vi "抽样与分割 - 副本.vi"(4 "stop (F)":bool caption="停止(F)", 8 "采样数":i32, 9 "采样率":i32[](array[numeric])=[32000, 32000, 32000, 32000, 32000, 32000, 80000, 80000], 10 "6133队列":refnum<queue>, 11 "数据队列":refnum<queue>) -> ()   [LabVIEW 2014]
panel:
  in  "发送次数":i32=1
  out "每通道发送的数据量":i32[](array[numeric])
  in  "读取次数":dbl=1.0
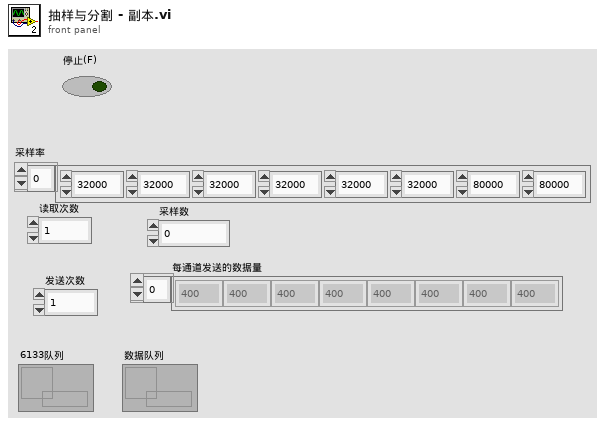
[diagram p1: front panel]
types:
  T1 = cluster{"设备名":string, "时间":timestamp, "数据":sgl[][]}
  T2 = cluster{"设备名":string, "时间":timestamp, "输出数组":dbl[][], "每通道发送的数据量":i32[], i32}
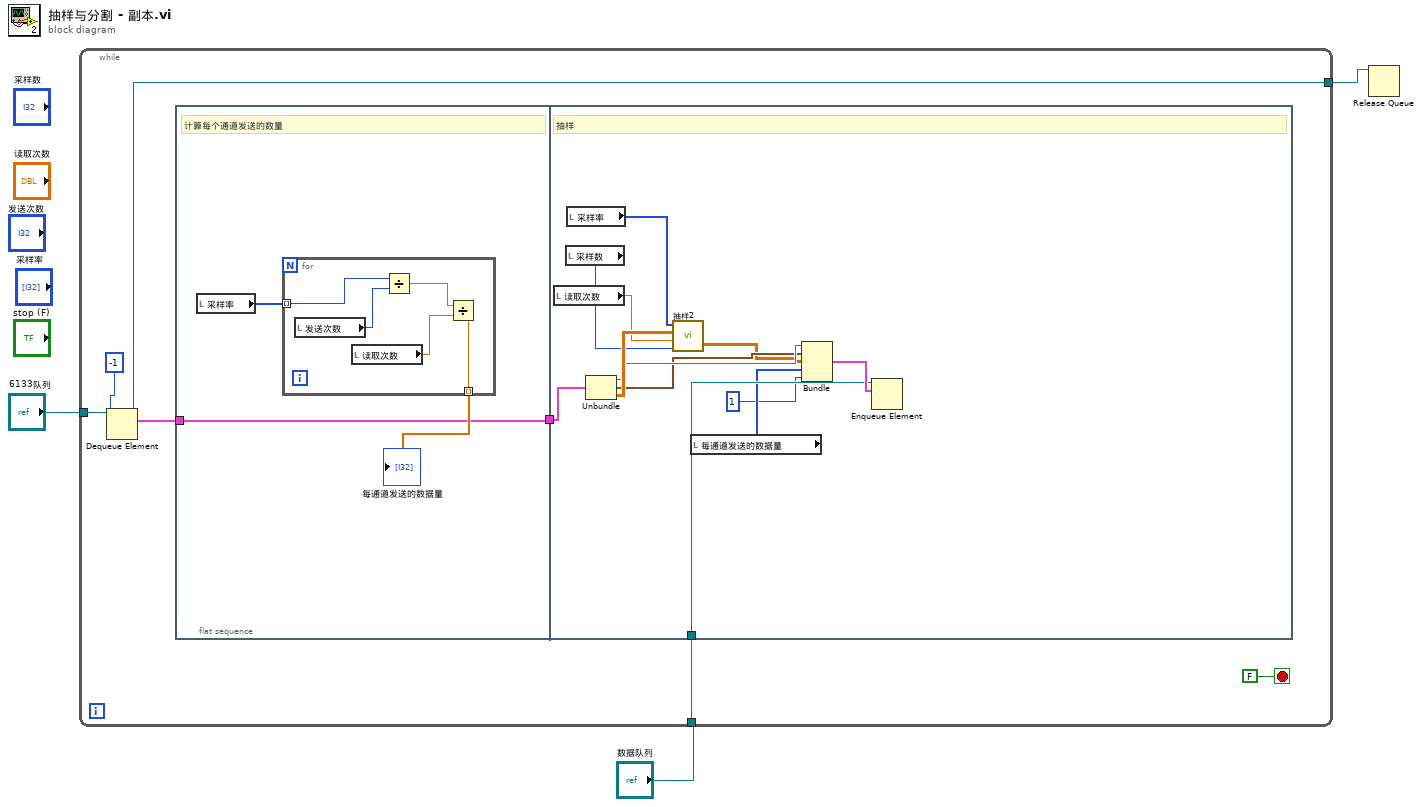
[diagram p0: block diagram]
diagram:
  n1 = while "While循环" {
    tunnel: "6133队列" -> [w10]
    tunnel: [w9] -> w2
    tunnel: "数据队列" -> [w4]
    stop <- FALSE stop-if-true
    n2 = Dequeue Element(queue=w10, timeout in ms (-1)=-1 ("超时毫秒(-1)")) -> (queue out=w9:refnum<queue>, element=w7:T1)  [unwired: 1 in, 2 out]
    n3 = flat-sequence "平铺式顺序结构" {
      tunnel: [w11] -> w6
      tunnel: w7 -> [w11]
      tunnel: w6 -> [w30]
      tunnel: w4 -> [w24]
      frame #0 {
        # "计算每个通道发送的数量"
        n4 = local read "采样率"() -> (w13:i32[])
        n5 = for "For循环" {
          tunnel: w13 -> [w15] mode=indexing
          tunnel: [w14] -> w12 mode=indexing
          n6 = local read "发送次数"() -> (w16:i32)
          n7 = local read "读取次数"() -> (w18:dbl)
          n8 = Divide(x=w15, y=w16) -> (x/y=w17:dbl)
          n9 = Divide(x=w17, y=w18) -> (x/y=w14:dbl)
        }
        "每通道发送的数据量" <- w12
      }
      frame #1 {
        # "抽样"
        n10 = local read "读取次数"() -> (w27:dbl)
        n11 = local read "采样数"() -> (w28:i32)
        n12 = local read "采样率"() -> (w26:i32[])
        n13 = Unbundle(w30) -> ("设备名"=w23:string, "时间"=w22:timestamp, "数据"=w29:sgl[][])
        n14 = call "抽样2.vi"("采样数"=w28, "读取次数"=w27, "采集数据"=w29, "采样率"=w26) -> ("输出数组"=w21:dbl[][])  [unwired: 1 out]
        n15 = local read "每通道发送的数据量"() -> (w20:i32[])
        n16 = Bundle("设备名"=w23, "时间"=w22, "输出数组"=w21, "每通道发送的数据量"=w20, 1) -> (w25:T2)  [unwired: 1 in]
        n17 = Enqueue Element(queue=w24, element=w25) -> ()  [unwired: 2 in, 3 out]
      }
    }
  }
  n18 = Release Queue(queue=w2) -> ()  [unwired: 2 in, 3 out]
